vi "Autotest_Instr.vi"(8 "error in (no error)":errorcluster caption="entrée d'erreur (pas d'erreur)", 11 "Class DIO en entrée":refnum<class "Class Instrument DIO.lvclass">) -> (0 "error out":errorcluster caption="sortie d'erreur", 3 "Class DIO en Sortie":refnum<class "Class Instrument DIO.lvclass">)   [LabVIEW 2020, in "Library Instrument & Equipement.lvlib" / "Library Instruments.lvlib" / "Class Instrument DIO.lvclass"]
uses:
  Class Instrument DIO.lvclass
  C:/Users/ngarcin/OneDrive - Altyor/Standard TB/Class/Instrument/Instrument (Default)/Class Instrument (Default).lvclass
  Class Instrument DIO.lvclass/Class Instrument DIO.ctl
  Instrument (Default)/Class Instrument (Default).lvclass
  DIO/Class DIO (Default)/Class DIO (Default).lvclass
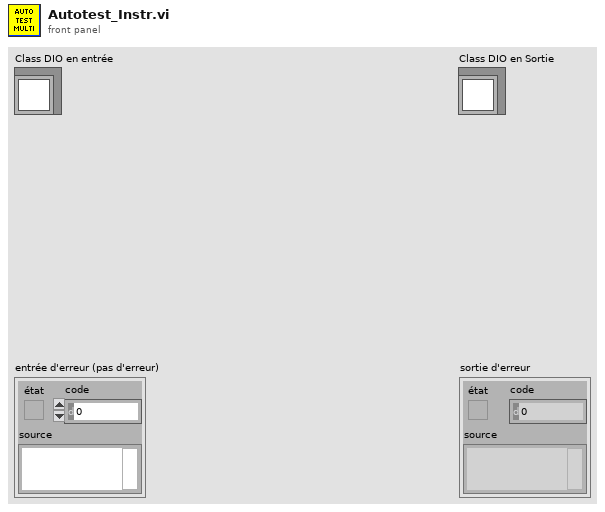
[diagram p1: front panel]
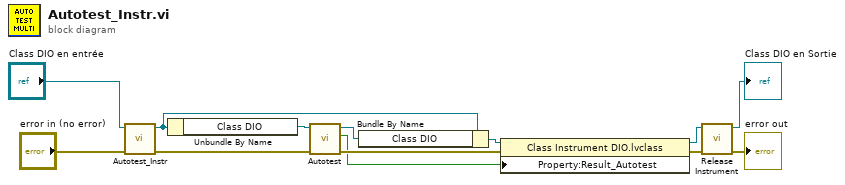
[diagram p0: block diagram]
diagram:
  n1 = call-parent "Autotest_Instr.vi"("error in (no error)"="error in (no error)", "Class Instrument (Default) en entrée"="Class DIO en entrée") -> ("error out"=w5:errorcluster, "Class Instrument (Default) en sortie"=w11:refnum<class "Class Instrument DIO.lvclass">)  [unwired: 8 in]
  n2 = Unbundle By Name(w11) -> ("Class DIO"=w3:refnum<class "Class DIO (Default).lvclass">)
  n3 = call-dynamic "Autotest.vi"("error in (no error)"=w5, "Class DIO (Default) en entrée"=w3) -> ("error out"=w4:errorcluster, "Autotest Ok"=w1:bool, "Class DIO (Default) en sortie"=w2:refnum<class "Class DIO (Default).lvclass">)  [unwired: 7 in]
  n4 = Bundle By Name(cluster=w11, "Class DIO"=w2) -> (w10:refnum<class "Class Instrument DIO.lvclass">)
  n5 = property class="Class Instrument DIO.lvclass"(reference=w10, error in=w4, "Property:Result_Autotest"=w1) -> (reference out=w7:refnum<class "Class Instrument DIO.lvclass">, error out=w9:errorcluster)
  n6 = call-dynamic "Release Instrument.vi"("error in (no error)"=w9, "Class Instrument (Default) en entrée"=w7) -> ("error out"=→"error out":errorcluster, "Class Instrument (Default) en sortie"=→"Class DIO en Sortie":refnum<class "Class Instrument DIO.lvclass">)  [unwired: 8 in]
